vi "CreateCopyExactPackage.vi"(8 "Error In":errorcluster, 9 "Reference Package Versions (Optional)":string[][](table), 10 "Package Suffix":string="CE", 11 "Package Path":path) -> (0 "Error Out":errorcluster, 1 "Ignored Dependencies":string[](array[string]), 2 "Copy Exact Dependencies":string[](array[string]), 3 "Copy Exact Package Path":path)   [LabVIEW 2019, in "CEPM.lvlib"]
uses:
  CEPM.lvlib
  <vilib>/National Instruments/NIPM API (Beta)/NIPM_API.lvlib
  <vilib>/SLL Toolkit/SLL File IO/SLL File IO.lvlib
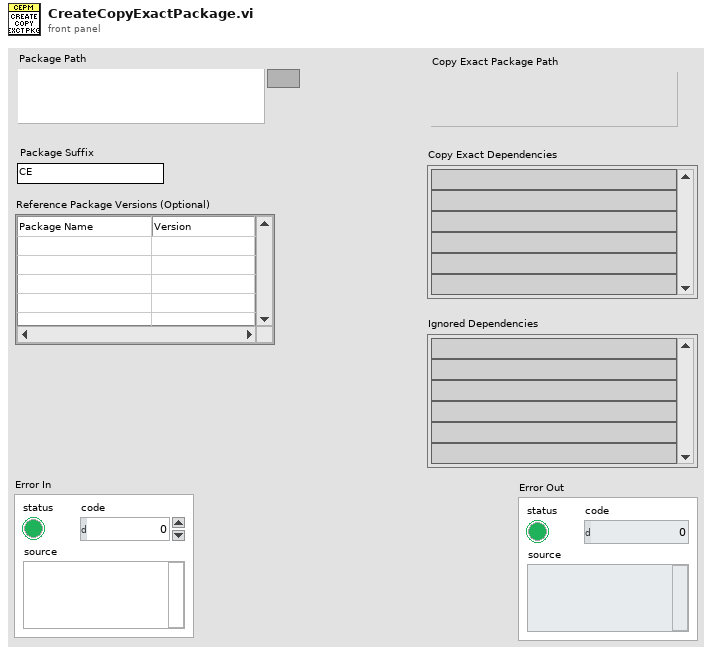
[diagram p1: front panel]
types:
  T1 = typedef "NIPM_API.lvlib/package attributes.ctl" = cluster{"Package Name":string, "Display name":string, "Version":string, "Display version":string, "Synopsis":string, "Description":string, "Maintainer":string, "Maintainer email address":string, "Category":string, "Homepage":string, "Release notes":string, "Depends":string[], "Recommends":string[], "Suggests":string[], "Conflicts":string[], "Provides":string[], "Replaces":string[], "Supplements":string[], "Enhances":string[], "Product":bool, "User visible":bool, "Installed size (KB)":u64, "Package filesize (bytes)":u64, "Architecture":string, "Agent":string, "MD5Checksum":string}
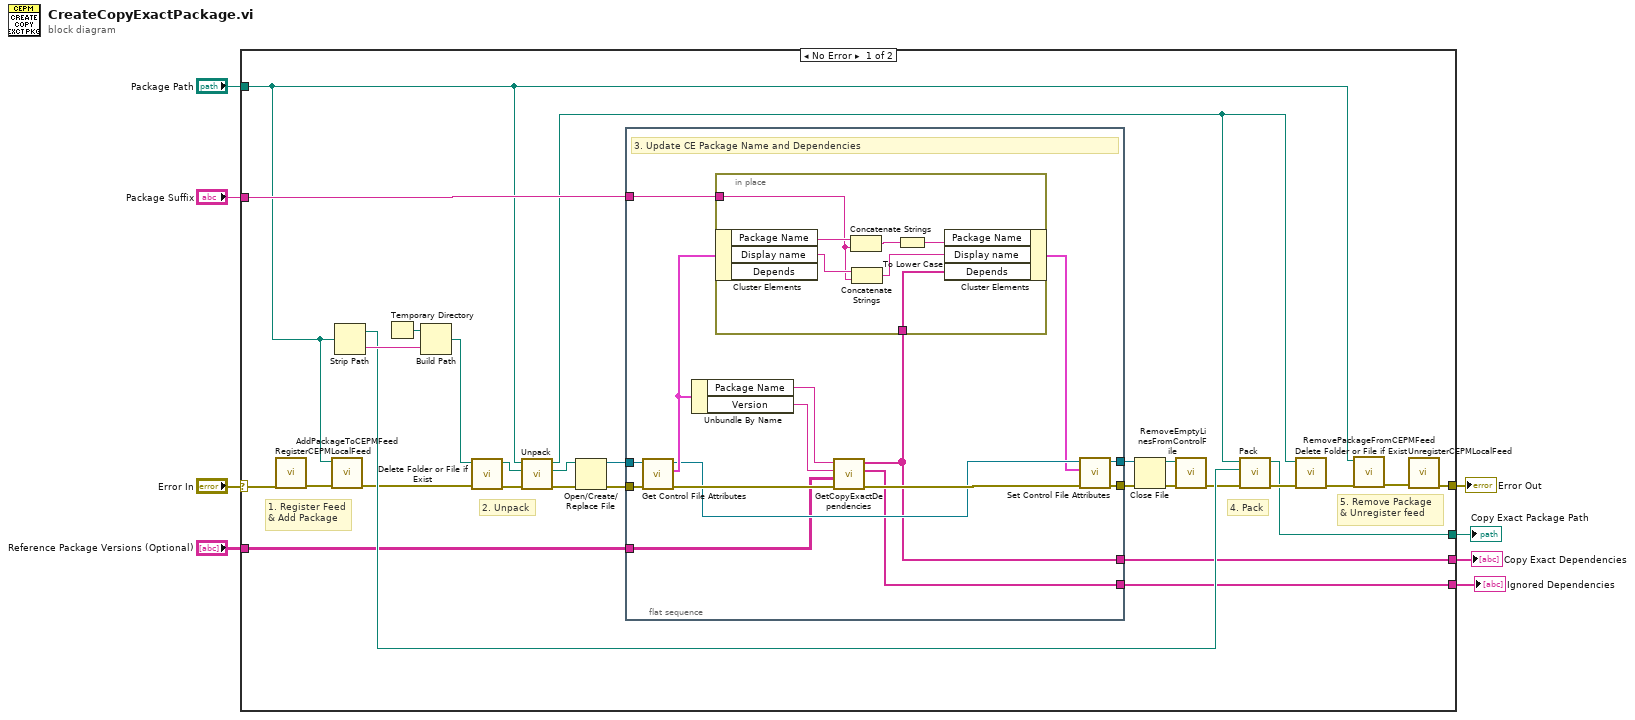
[diagram p0: block diagram]
diagram:
  n1 = case shown="No Error" "Error In" {
    selector: "Error In" -> [w16 w60]
    tunnel: "Package Path" -> [w10 _]
    tunnel: "Package Suffix" -> [w28 _]
    tunnel: [w11 w60] -> w5
    tunnel: "Reference Package Versions (Optional)" -> [w19 _]
    tunnel: [w18 _] -> w3
    tunnel: [w17 _] -> w2
    tunnel: [w9 _] -> w1
    frame No Error {
      # "5. Remove Package\n& Unregister feed"
      # "4. Pack"
      # "2. Unpack"
      # "1. Register Feed\n& Add Package"
      n2 = call "RegisterCEPMLocalFeed.vi"("Error In"=w16) -> ("Error Out"=w15:errorcluster)  [unwired: 10 in]
      n3 = call "AddPackageToCEPMFeed.vi"("Error In"=w15, "Package Path"=w10) -> ("Error Out"=w14:errorcluster)  [unwired: 9 in]
      n4 = Strip Path(path=w10) -> (stripped path=w26:path, name=w32:string)
      n5 = Temporary Directory() -> (w33:path)
      n6 = Build Path(base path=w33, name or relative path=w32) -> (appended path=w31:path)
      n7 = call <vilib>:"Delete Folder or File if Exist.vi"("error in (no error)"=w14, "Path"=w31) -> ("error out"=w29:errorcluster, "Path out"=w30:path)  [unwired: 8 in]
      n8 = call <vilib>:"Unpack.vi"("error in"=w29, "destination folder"=w30, "nipkg filepath"=w10) -> ("error out"=w34:errorcluster, "control filepath"=w35:path, "unpacked folderpath"=w20:path)  [unwired: 4 in, 2 out]
      n9 = Open/Create/Replace File(file path (use dialog)=w35, error in=w34) -> (refnum out=w36:refnum<file>, error out=w37:errorcluster)  [unwired: 4 in, 1 out]
      n10 = flat-sequence {
        tunnel: w37 -> [w52]
        tunnel: w36 -> [w51]
        tunnel: w28 -> [w45]
        tunnel: [w44] -> w27
        tunnel: [w41] -> w25
        tunnel: w19 -> [w40]
        tunnel: [w39] -> w17
        tunnel: [w38] -> w9
        frame #0 {
          # "3. Update CE Package Name and Dependencies"
          n11 = call <vilib>:"Get Control File Attributes.vi"("error in (no error)"=w52, "control file refnum in"=w51) -> ("error out"=w49:errorcluster, "package attributes"=w46:T1, "control file refnum out"=w43:refnum<file>)  [unwired: 7 in]
          n12 = Unbundle By Name(w46) -> ("Package Name"=w50:string, "Version"=w47:string)
          n13 = call "GetCopyExactDependencies.vi"("Error In"=w49, "Reference Package Versions (Optional)"=w40, "Package Version"=w47, "Package Name"=w50) -> ("Error Out"=w48:errorcluster, "Ignored Dependencies"=w38:string[], "Copy Exact Dependencies"=w39:string[])  [unwired: 5 in]
          n14 = in-place {
            in-place-border: w45 -> [w57]
            in-place-border: w39 -> [w54]
            n15 = in-place-cluster #1(w46) -> ("Package Name"=w59:string, "Display name"=w58:string)  [unwired: 1 out]
            n16 = Concatenate Strings(w59, w57) -> (w53:string)
            n17 = Concatenate Strings(w58, w57) -> (w56:string)
            n18 = To Lower Case(string=w53) -> (all lower case string=w55:string)
            n19 = in-place-cluster #1("Package Name"=w55, "Display name"=w56, "Depends"=w54) -> (w42:T1)
          }
          n20 = call <vilib>:"Set Control File Attributes.vi"("error in (no error)"=w48, "package attributes"=w42, "control file refnum in"=w43) -> ("error out"=w44:errorcluster, "control file refnum out"=w41:refnum<file>)  [unwired: 7 in]
        }
      }
      n21 = Close File(refnum=w25, error in=w27) -> (path=w22:path, error out=w24:errorcluster)
      n22 = call "RemoveEmptyLinesFromControlFile.vi"("Error In"=w24, "Control File Path"=w22) -> ("Error Out"=w23:errorcluster)  [unwired: 9 in]
      n23 = call <vilib>:"Pack.vi"("error in"=w23, "destination folder"=w26, "source folder"=w20) -> ("error out"=w21:errorcluster, "package filepath"=w18:path)  [unwired: 7 in]
      n24 = call <vilib>:"Delete Folder or File if Exist.vi"("error in (no error)"=w21, "Path"=w20) -> ("error out"=w13:errorcluster)  [unwired: 8 in, 1 out]
      n25 = call "RemovePackageFromCEPMFeed.vi"("Error In"=w13, "Package Path"=w10) -> ("Error Out"=w12:errorcluster)  [unwired: 9 in]
      n26 = call "UnregisterCEPMLocalFeed.vi"("Error In"=w12) -> ("Error Out"=w11:errorcluster)  [unwired: 10 in]
    }
    frame Error {
    }
  }
  "Error Out" <- w5
  "Copy Exact Dependencies" <- w2
  "Copy Exact Package Path" <- w3
  "Ignored Dependencies" <- w1
